vi "TestFileInterface.vi"() -> ()   [LabVIEW 2020]
uses:
  <vilib>/NI/NI VeriStand Advanced SysDef API/_Types/SysDef.Export.ctl
  <vilib>/NI/NI VeriStand Advanced SysDef API/_Types/TreeItem.ctl
  <vilib>/NI/NI VeriStand Advanced SysDef API/_Types/TreeItem.Info.ctl
  <vilib>/NI VeriStand/Custom Device API/Custom Device Channel.ctl
  <vilib>/NI VeriStand/Custom Device API/Custom Device Channel Type.ctl
  <vilib>/NI VeriStand/Custom Device API/Custom Device Waveform.ctl
  <vilib>/NI VeriStand/Custom Device API/Custom Device Waveform DataType.ctl
  <vilib>/NI/NI VeriStand Advanced SysDef API/_Types/TreeItem.Property.ctl
  Source/Section File Interface Class/Section File Interface.lvclass
  C:/git/fmussi_niveristand-custom-device-development-tools/import-export/Source/File Interface Class/File Interface.lvclass
  Source/File Interface Class/File Interface.lvclass
  <vilib>/NI/NI VeriStand Advanced SysDef API/SysDef API/Advanced System Definition.lvlib
  <vilib>/NI VeriStand/Custom Device API/Custom Device API.lvlib
panel:
  in  "Boolean":bool
  in  "ImportExport.lvlib:File Interface.lvclass":refnum<class "File Interface.lvclass">
  in  "ImportExport.lvlib:Section File Interface.lvclass":refnum<class "Section File Interface.lvclass">
  out "SysDef":T1 {"Tree"."Properties"."Type" items=["K_STRING", "K_BOOL", "K_I32", "K_U32", "K_DOUBLE", "K_U64", "K_VARIANT", "K_DEPENDENTFILE", "K_DEPENDENTNODE", "K_DATASOURCENODE", "K_U16", "K_DBLARR", "K_U32ARR", "K_I32ARR", "K_STRINGARR", "K_DICTIONARY", "K_DICTIONARYARR"]}
  in  "Path":path
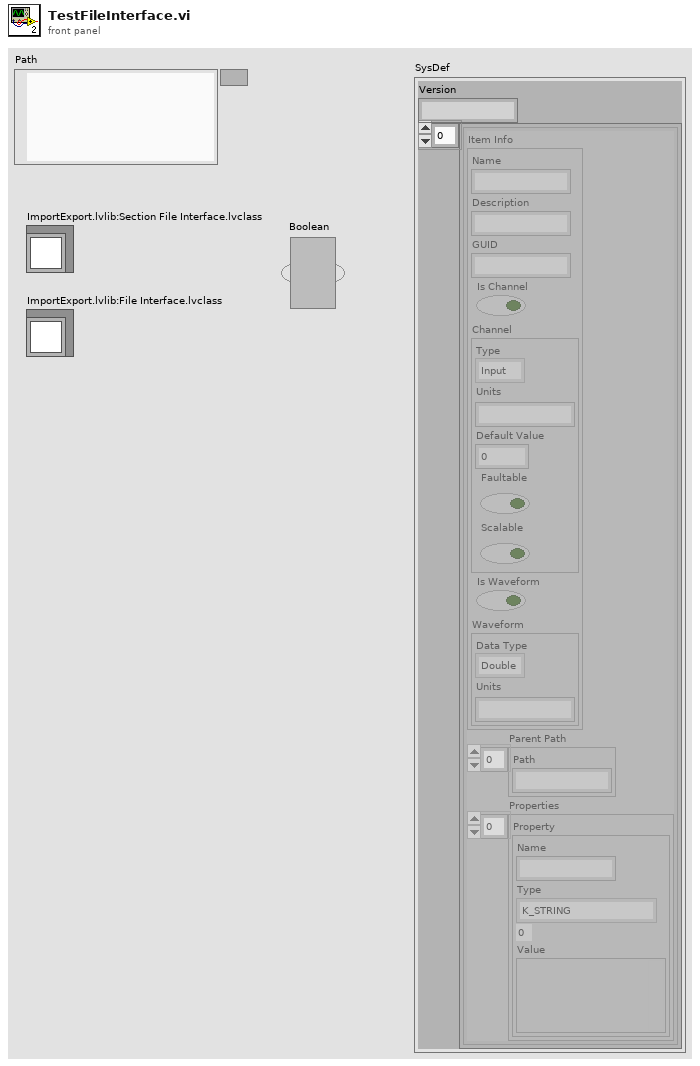
[diagram p1: front panel]
types:
  T1 = typedef "Advanced System Definition.lvlib/SysDef.Export.ctl" = cluster{"Version":string, "Tree":T2[]}
  T2 = typedef "Advanced System Definition.lvlib/TreeItem.ctl" = cluster{"Item Info":T3, "Parent Path":string[], "Properties":T8[]}
  T3 = typedef "Advanced System Definition.lvlib/TreeItem.Info.ctl" = cluster{"Name":string, "Description":string, "GUID":string, "Is Channel":bool, "Channel":T4, "Is Waveform":bool, "Waveform":T6}
  T4 = typedef "Custom Device API.lvlib/Custom Device Channel.ctl" = cluster{"Type":T5, "Units":string, "Default Value":dbl, "Faultable":bool, "Scalable":bool}
  T5 = typedef "Custom Device API.lvlib/Custom Device Channel Type.ctl" = enum16{"Input", "Output"}
  T6 = typedef "Custom Device API.lvlib/Custom Device Waveform.ctl" = cluster{"Data Type":T7, "Units":string}
  T7 = typedef "Custom Device API.lvlib/Custom Device Waveform DataType.ctl" = enum16{"Double", "Complex Double"}
  T8 = typedef "Advanced System Definition.lvlib/TreeItem.Property.ctl" = cluster{"Name":string, "Type":i32, "Value":variant}
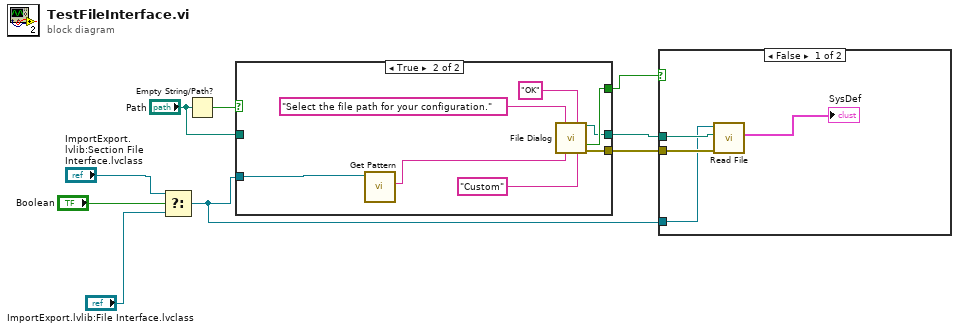
[diagram p0: block diagram]
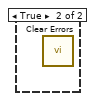
[diagram p2: hidden frame]
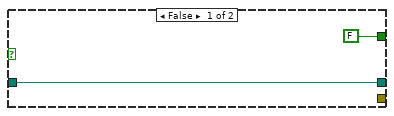
[diagram p3: hidden frame]
diagram:
  n1 = Select(t="ImportExport.lvlib:Section File Interface.lvclass", s="Boolean", f="ImportExport.lvlib:File Interface.lvclass") -> (s? t:f=w1:refnum<class "File Interface.lvclass">)
  n2 = Empty String/Path?(string/path="Path") -> (empty?=w9:bool)
  n3 = case shown="True" w9 {
    tunnel: [FALSE ("cancelled") w16] -> w7
    tunnel: [_ w15] -> w6
    tunnel: [w10 w12] -> w5
    tunnel: w1 -> [_ w14]
    tunnel: "Path" -> [w10 _]
    frame False {
    }
    frame True {
      n4 = call-dynamic "Get Pattern.vi"("File Interface in"=w14) -> ("file extension"=w13:string)  [unwired: 10 in]
      n5 = call "File Dialog"("prompt"="Select the file path for your configuration.", "button label"="OK", "pattern (all files)"=w13, "pattern label"="Custom") -> ("selected path"=w12:path, "cancelled"=w16:bool, "error out"=w15:errorcluster)  [unwired: 8 in, 1 out]
    }
  }
  n6 = case shown="False" w7 {
    tunnel: w6 -> [w23 _]
    tunnel: w5 -> [w22 _]
    tunnel: w1 -> [w20 _]
    frame False {
      n7 = call-dynamic "Read File.vi"("error in (no error)"=w23, "Path in"=w22, "File Interface in"=w20) -> ("SysDef"=→"SysDef":T1)  [unwired: 7 in, 1 out]
    }
    frame True {
      n8 = call <vilib>:"Clear Errors.vi"() -> ()  [unwired: 6 in, 2 out]
    }
  }
